vi "Command_Joint_Angles.vi"(0 "Side":T3, 1 "node":string, 2 "Arm Angles (degrees)":T2, 3 "error in":errorcluster, 4 "Mode":T1=1 items=["Position"=1, "Velocity"=2, "Effort"=3]) -> (6 "error out":errorcluster)   [LabVIEW 2012]
doc: "Set joints on Baxter's right or left side by position, velocity, or effort"
uses:
  <userlib>/ROSforLV/ROS/Code/SubVIs/BaxterSide.ctl
  <userlib>/ROSforLV/ROS/Code/SubVIs/BaxterArmsSmall.ctl
  <userlib>/ROSforLV/ROS/Code/SubVIs/JointMode.ctl
  <userlib>/ROSforLV/ROS/Code/Console/Servers/ServerSubs/TopicDef.ctl
  <userlib>/ROSforLV/ROS/Code/SubVIs/_ROSDirection.ctl
panel:
  out "Move Command":string
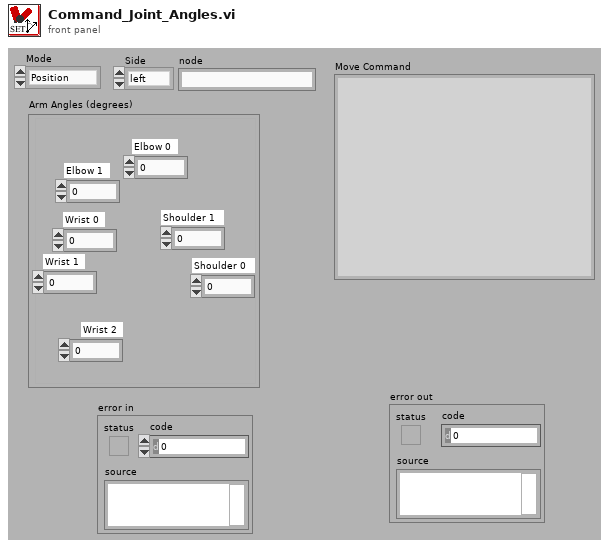
[diagram p1: front panel]
types:
  T1 = typedef "JointMode.ctl" = u8
  T2 = typedef "BaxterArmsSmall.ctl" = cluster{"Elbow 0":dbl, "Elbow 1":dbl, "Shoulder 0":dbl, "Shoulder 1":dbl, "Wrist 0":dbl, "Wrist 1":dbl, "Wrist 2":dbl}
  T3 = typedef "BaxterSide.ctl" = enum16{"left", "right"}
  T4 = typedef "TopicDef.ctl" = cluster{"Topic":string, "Type":string, "Action":T5, "Update (ms)":u16, "queue size":u16}
  T5 = typedef "_ROSDirection.ctl" = enum16{"Node", "Publisher", "Subscriber", "Service Client"}
  T6 = typedef "_ROSControl.ctl" = cluster{"topic port":u16, "Node":string, "topic":string, "type":string, "node port":u16, "error ":errorcluster, "Direction":T5, "Update (ms)":u16, "queue size":u16}
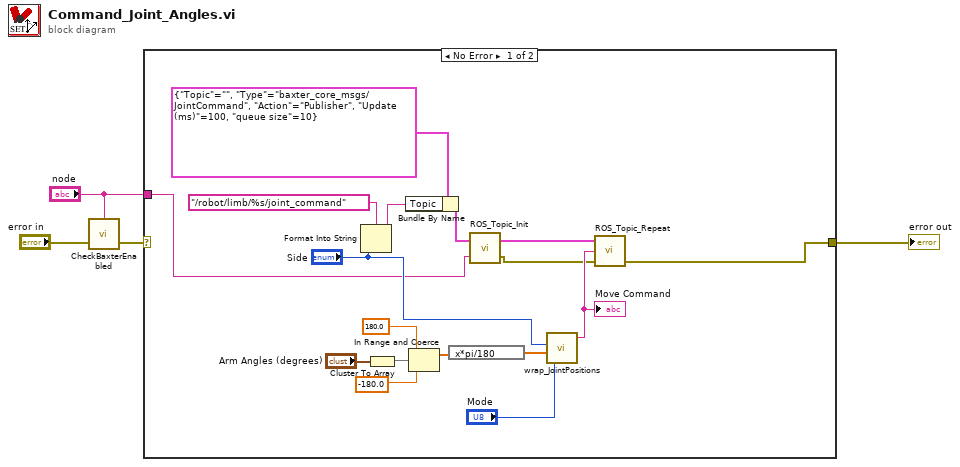
[diagram p0: block diagram]
diagram:
  n1 = call <userlib>:"CheckBaxterEnabled.vi"("error in"="error in", "node"="node") -> ("error out"=w2:errorcluster)  [unwired: 2 in]
  n2 = case shown="No Error" w2 {
    selector: w2 -> [_ w22]
    tunnel: [w5 w22] -> w4
    tunnel: "node" -> [w8 _]
    frame No Error {
      n3 = Format Into String(format string="/robot/limb/%s/joint_command" ("Topic"), "Side") -> (resulting string=w12:string)  [unwired: 2 in, 1 out]
      n4 = Cluster To Array(cluster="Arm Angles (degrees)") -> (array=w19:dbl[])
      n5 = Bundle By Name(cluster=T4 {"Topic"="", "Type"="baxter_core_msgs/JointCommand", "Action"=enum."Publisher", "Update (ms)"=100, "queue size"=10} ("Definitions"), "Topic"=w12) -> (w9:T4)
      n6 = In Range and Coerce(upper limit=180.0 ("Elbow 0"), x=w19, lower limit=-180.0 ("Elbow 0")) -> (coerced(x)=w16:dbl[])  [unwired: 1 out]
      n7 = expression code="x*pi/180"(w16) -> (w15:dbl[])
      n8 = call <userlib>:"ROS_Topic_Init.vi"("node"=w8, "Definitions"=w9) -> ("error out"=w6:errorcluster, "ROS out"=w21:T6)
      n9 = call <userlib>:"wrap_JointPositions.vi"("Mode"="Mode", "Positions"=w15, "Side"="Side") -> ("msg out"=w7:string)  [unwired: 3 in]
      "Move Command" <- w7
      n10 = call <userlib>:"ROS_Topic_Repeat.vi"("error in (no error)"=w6, "Msg in"=w7, "ROS in"=w21) -> ("error out"=w5:errorcluster)  [unwired: 1 in, 1 out]
    }
    frame Error {
    }
  }
  "error out" <- w4
